vi "Charge Model.vi"(0 "Rated Capacity (AH)":dbl=100.0, 5 "Charge Current (A)":dbl=1.0, 7 "Cell Voltage (V)":dbl=3.2, 9 "Sample Rate (Hz)":i32=1000) -> (6 "Cell Voltage (V)":dbl[](array[numeric]), 8 "Cell Current (A)":dbl[](array[numeric]), 10 "SoC (%)":dbl[](array[numeric]))   [LabVIEW 2023]
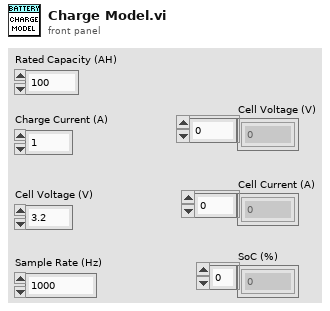
[diagram p1: front panel]
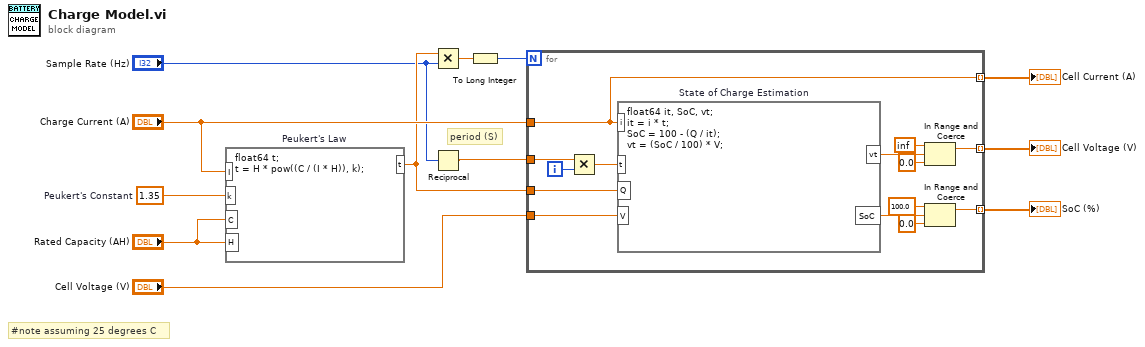
[diagram p0: block diagram]
diagram:
  w11 = 1.35  # Peukert's Constant
  # "period (S)"
  # "#note assuming 25 degrees C"
  n1 = formula code="float64 t;\nt = H * pow((C / (I * H)), k);" "Peukert's Law"("k"=w11, "C"="Rated Capacity (AH)", "I"="Charge Current (A)", "H"="Rated Capacity (AH)") -> ("t"=w6:dbl)
  n2 = Multiply(x=w6, y="Sample Rate (Hz)") -> (x*y=w3:dbl)
  n3 = Reciprocal(x="Sample Rate (Hz)") -> (1/x=w4:dbl)
  n4 = To Long Integer(number=w3) -> (32bit integer=w2:i32)
  n5 = for {
    N: w2 -> [_]
    tunnel: w6 -> [w26]
    tunnel: "Charge Current (A)" -> [w17]
    tunnel: "Cell Voltage (V)" -> [w25]
    tunnel: [w17] -> w8 mode=indexing
    tunnel: [w16] -> w1 mode=indexing
    tunnel: [w15] -> w7 mode=indexing
    tunnel: w4 -> [w13]
    i -> [w14]
    n6 = Multiply(x=w13, y=w14) -> (x*y=w18:dbl)
    n7 = formula code="float64 it, SoC, vt;\nit = i * t;\nSoC = 100 - (Q / it);\nvt = (SoC / 100) * V;" "State of Charge Estimation"("Q"=w26, "i"=w17, "t"=w18, "V"=w25) -> ("SoC"=w20:dbl, "vt"=w24:dbl)
    n8 = In Range and Coerce(upper limit=inf, x=w24, lower limit=0.0) -> (coerced(x)=w16:dbl)  [unwired: 1 out]
    n9 = In Range and Coerce(upper limit=100.0, x=w20, lower limit=0.0) -> (coerced(x)=w15:dbl)  [unwired: 1 out]
  }
  "Cell Current (A)" <- w8
  "Cell Voltage (V)" <- w1
  "SoC (%)" <- w7
